vi "DSP_tester.vi"() -> ()   [LabVIEW 2021]
uses:
  <instrlib>/_niInstr/DSP/v1/Shared/Public/IQ Data.ctl
  <instrlib>/_niInstr/DSP/v1/FPGA/Public/Sub VIs/Data Conversion/U32 to IQ - 1 spc - S18.1.vi
  <instrlib>/_niInstr/Basic Elements/v1/FPGA/Private/Count Up U8.vi
  <instrlib>/_niInstr/DSP/v1/FPGA/niInstr DSP v1 FPGA.lvlib
  <instrlib>/_niInstr/DSP/v1/Shared/niInstr DSP v1 Shared.lvlib
  <instrlib>/_niInstr/Basic Elements/v1/FPGA/niInstr Basic Elements v1 FPGA.lvlib
panel:
  out "Waveform Chart 2":dbl(graph)
  out "Numeric":i32
  out "count out":u8
  in  "output sample rate":dbl format="%#1.5p"
  in  "f shift":dbl format="%#_6p"
  in  "ftest":dbl format="%#_6p"
  in  "Stop":bool
  out "Waveform Chart":dbl(graph)
  in  "reset":bool
  in  "Cluster":T1 {"frequency shift" format="%#.48g"}
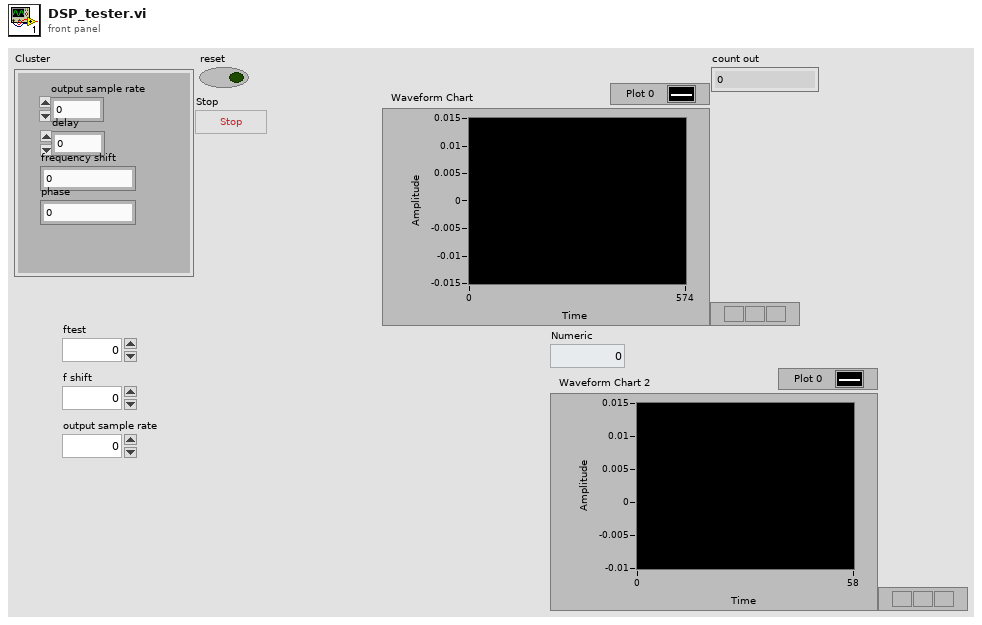
[diagram p1: front panel]
types:
  T1 = cluster{"output sample rate":fxp<+,48,1>, "delay":fxp<+/-,16,0>, "frequency shift":fxp<+/-,48,0>, "phase":fxp<+/-,21,0>}
  T2 = typedef "niInstr DSP v1 Shared.lvlib/IQ Data.ctl" = cluster{"I":fxp<+/-,18,1>, "Q":fxp<+/-,18,1>, "overflow":bool}
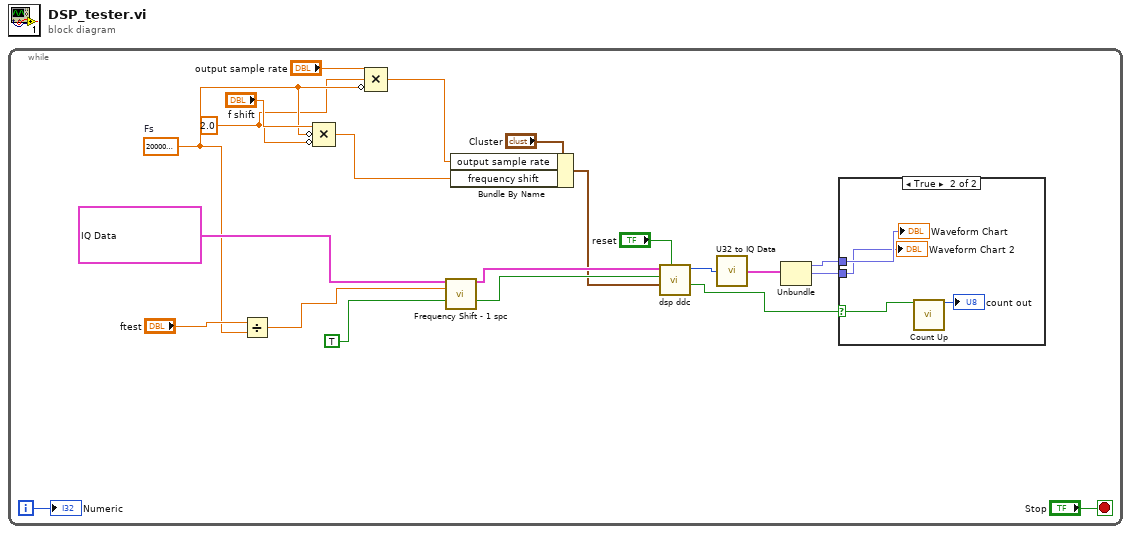
[diagram p0: block diagram]
diagram:
  n1 = while {
    i -> [w2]
    stop <- "Stop" stop-if-true
    w4 = 2.0 ("value")
    w5 = 200000000.0  # Fs
    n2 = Divide(x="ftest", y=w5) -> (x/y=w10:dbl)
    n3 = Compound Arithmetic op=MULTIPLY("f shift", invert w5, invert w4) -> (w9:dbl)
    n4 = Compound Arithmetic op=MULTIPLY("output sample rate", w4, invert w5) -> (w6:dbl)
    n5 = call <instrlib>:"Frequency Shift - 1 spc.vi"("data in"=T2 {"I"=0.01000213623046875, "Q"=0.0, "overflow"=FALSE}, "frequency shift"=w10, "input valid"=TRUE) -> ("data out"=w22:T2, "output valid"=w19:bool)  [unwired: 9 in, 2 out]
    n6 = Bundle By Name(cluster="Cluster", "output sample rate"=w6, "frequency shift"=w9) -> (w12:T1)
    n7 = call "dsp ddc.vi"("reset"="reset", "Cluster"=w12, "input valid"=w19, "data in"=w22) -> ("output valid"=w3:bool, "data out"=w17:u32)  [unwired: 5 in, 1 out]
    n8 = call-poly <instrlib>:"U32 to IQ Data.vi"("U32 data"=w17) -> ("IQ data"=w16:T2)  [unwired: 14 in]
    n9 = Unbundle(w16) -> ("I"=w15:fxp<+/-,18,1>, "Q"=w1:fxp<+/-,18,1>)  [unwired: 1 out]
    n10 = case shown="True" w3 {
      selector: w3 -> [_ w25]
      tunnel: w15 -> [_ w26]
      tunnel: w1 -> [_ w23]
      frame False {
      }
      frame True {
        n11 = call-poly <instrlib>:"Count Up.vi"("increment"=w25) -> ("count out"=→"count out":u8)  [unwired: 14 in]
        "Waveform Chart" <- w26
        "Waveform Chart 2" <- w23
      }
    }
    "Numeric" <- w2
  }
